vi "TEST_bench_FXP_Nbarr_re_Kx_singleAxis.vi"(6 "NS + 1":u8=9, 8 "K_lqr":fxp<+/-,32,15>[](array[numeric])=[0.0, 0.0, 0.0, 0.0, 0.0, 0.0, 0.0, 0.0, 0.0, 0.0, 0.0, 0.0, 0.0, 0.0, 0.0, 0.0, 0.0, 0.0, 0.0, 0.0, 0.0, 0.0, 0.0, 0.0, 0.0, 0.0, 0.0, 0.0, 0.0, 0.0, 0.0, 0.0, 0.0, 0.0, 0.0, 0.0, 0.0, 0.0, 0.0, 0.0, 0.0, 0.0, 0.0, 0.0, 0.0, 0.0, 0.0, 0.0, 0.0, 0.0]) -> (1 "del u_x":fxp<+/-,64,15>)   [LabVIEW 2017]
uses:
  fpga_subVIs_ssxy/fixed-point-ss/typeDefs/x_vec_type.ctl
  fpga_subVIs_ssxy/fixed-point-ss/typeDefs/Kz_bram.ctl
  fpga_subVIs_ssxy/fixed-point-ss/typeDefs/x_vec_bram.ctl
  <vilib>/rvi/Emulation/niFpgaEmulationIsFPGAContextNoSignature.vi
  <vilib>/rvi/DataTransferAndStorage/Container/Common/niFpgaContainerGetUniqueNameForEmu.vi
  <vilib>/rvi/Memory/Memory_Emulation/niFpgaMemoryEmulationCacheClearOnFirstRun.vi
  <vilib>/rvi/Memory/Memory_Emulation/nirvimemoryEmulationManagerCache_MakeExclusive.vi
  <vilib>/rvi/Memory/Memory_Emulation/niFpgaMemoryEmulationValidateCache.vi
  <vilib>/rvi/Memory/Memory_Emulation/nirvimemoryEmulationManagerCache_InsertValue.vi
  <vilib>/Utility/error.llb/Clear Errors.vi
  <vilib>/rvi/Memory/Memory_Emulation/nirvimemoryEmulationManagerCache_ReleaseExclusive.vi
  <vilib>/rvi/Memory/Memory_Emulation/nirvimemoryEmulationManagerCache_GetValue.vi
  <vilib>/rvi/Memory/Memory_Emulation/nirvimemoryEmulationManagerCache_SetValue.vi
  <vilib>/rvi/Emulation/niFpgaProcessEmulError.vi
  <vilib>/rvi/Emulation/niFpgaSctlEmulationGetInTimedLoop.vi
  <vilib>/rvi/DataTransferAndStorage/Container/Common/niFpgaContainerExecOnDevCompGetState.vi
  <vilib>/rvi/errors/nirviReportUnexpectedCaseInternalError (U32).vi
  <vilib>/rvi/Emulation/niFpgaSctlEmulationResourceMgr.vi
  <vilib>/rvi/DataTransferAndStorage/Container/XNode/niFpgaContainer.xnode
  <vilib>/rvi/DataTransferAndStorage/Register/Emulation/niFpgaRegisterEmulation.vi
  <vilib>/rvi/Memory/Memory_Emulation/niFpgaMemoryEmulationRefIn.vi
panel:
  in  "yd_est_x":fxp<+/-,32,5>
  in  "Nbar":fxp<+/-,32,5>
  in  "ref":fxp<+/-,32,5>
  in  "x_vec":T1=[0.0, 0.0, 0.0, 0.0, 0.0, 0.0, 0.0, 0.0, 0.0, 0.0, 0.0, 0.0, 0.0, 0.0, 0.0, 0.0, 0.0, 0.0, 0.0, 0.0, 0.0, 0.0, 0.0, 0.0, 0.0]
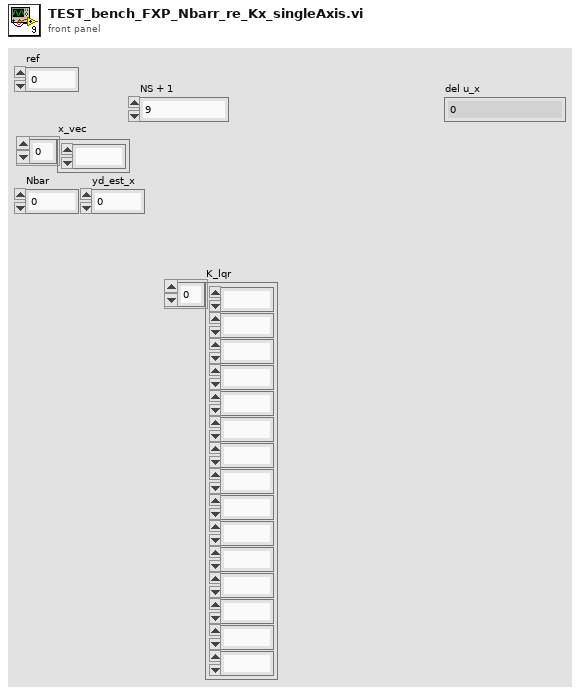
[diagram p1: front panel]
types:
  T1 = typedef "x_vec_type.ctl" = fxp<+/-,32,6>[]
  T2 = typedef "x_vec_bram.ctl" = refnum<k21>
  T3 = typedef "Kz_bram.ctl" = refnum<k21>
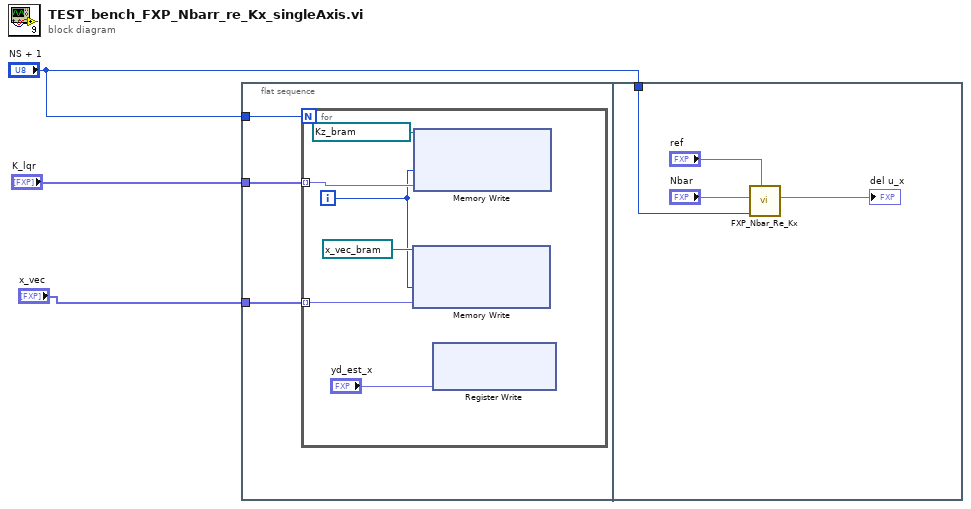
[diagram p0: block diagram]
diagram:
  n1 = flat-sequence {
    tunnel: "NS + 1" -> [w6]
    tunnel: "K_lqr" -> [w5]
    tunnel: "x_vec" -> [w4]
    tunnel: "NS + 1" -> [w16]
    frame #0 {
      n2 = for {
        N: w6 -> [_]
        tunnel: w5 -> [w12] mode=indexing
        tunnel: w4 -> [w8] mode=indexing
        i -> [w9]
        n3 = xnode "Memory Write"("Address"=w9, "Data"=w8, "Memory In"=T2 "xk_0_2" ("Memory")) -> ()  [unwired: 1 out]
        n4 = xnode "Memory Write"("Address"=w9, "Data"=w12, "Memory In"=T3 "K_FXP_row1" ("Memory")) -> ()  [unwired: 1 out]
        n5 = xnode "Register Write"("Data"="yd_est_x") -> ()  [unwired: 1 in, 1 out]
      }
    }
    frame #1 {
      n6 = call "FXP_Nbar_Re_Kx.vi"("ref"="ref", "NS"=w16, "Nbar"="Nbar") -> ("del u_x"=→"del u_x":fxp<+/-,32,16>)  [unwired: 8 in]
    }
  }
